vi "Flatten Value.vi"(8 "Error In":errorcluster, 11 "2D Int In":refnum<class "2D Int.lvclass">) -> (0 "Error Out":errorcluster, 1 "Value":string, 3 "2D Int Out":refnum<class "2D Int.lvclass">)   [LabVIEW 2017, in "Tree API.lvlib" / "2D Int.lvclass"]
doc: "Dynamic dispatch interface for flattening Tree Data classes to string."
uses:
  2D Int.lvclass
  Tree Manager/Tree.lvclass
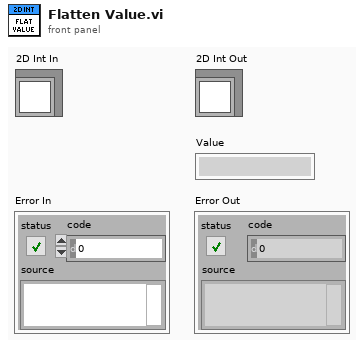
[diagram p1: front panel]
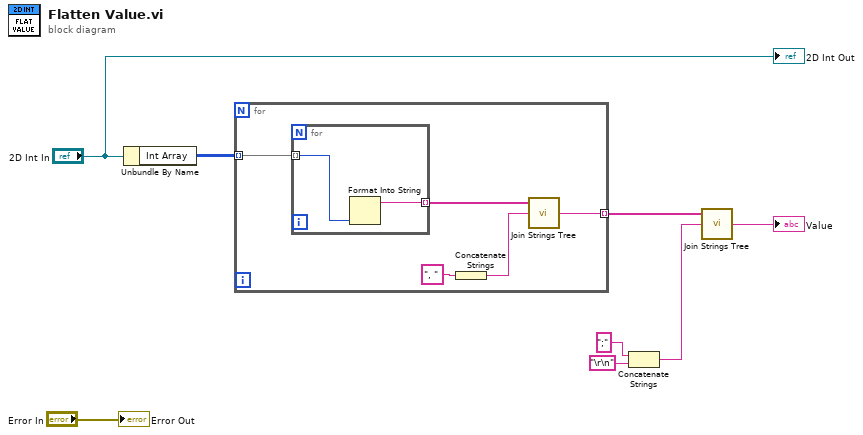
[diagram p0: block diagram]
diagram:
  n1 = Unbundle By Name("2D Int In") -> ("Int Array"=w5:i64[][])
  n2 = for {
    tunnel: w5 -> [w13] mode=indexing
    tunnel: [w11] -> w6 mode=indexing
    n3 = for {
      tunnel: w13 -> [w15] mode=indexing
      tunnel: [w14] -> w12 mode=indexing
      n4 = Format Into String(w15) -> (resulting string=w14:string)  [unwired: 3 in, 1 out]
    }
    n5 = Concatenate Strings(", " ("Separator (,)")) -> (w9:string)
    n6 = call "Join Strings Tree.vi"("Separator (,)"=w9, "Strings In"=w12) -> ("String"=w11:string)  [unwired: 1 in]
  }
  n7 = Concatenate Strings(";" ("Separator (,)"), "\r\n") -> (w2:string)
  n8 = call "Join Strings Tree.vi"("Separator (,)"=w2, "Strings In"=w6) -> ("String"=→"Value":string)  [unwired: 1 in]
  "2D Int Out" <- "2D Int In"
  "Error Out" <- "Error In"
